vi "lab7_task2.vi"() -> ()   [LabVIEW 2021]
uses:
  <vilib>/DAQmx/write.llb/DAQmx Write (Digital Bool 1Line 1Point).vi
  <vilib>/DAQmx/read.llb/DAQmx Read (Analog Wfm 1Chan NSamp).vi
  <vilib>/DAQmx/create/channels.llb/DAQmx Create Channel (AI-Voltage-Basic).vi
  <vilib>/DAQmx/configure/timing.llb/DAQmx Timing (Sample Clock).vi
  <vilib>/DAQmx/configure/trigger.llb/DAQmx Start Trigger (Digital Edge).vi
  <vilib>/DAQmx/miscellaneous.llb/DAQmx Fill In Error Info.vi
  <vilib>/DAQmx/create/channels.llb/DAQmx Create Channel (DO-Digital Output).vi
panel:
  in  "stop 2":bool
  in  "Trigger \nButton":bool
  in  "stop":bool
  in  "# samples to read":i32=1000
  out "Waveform Graph":waveform(dbl)(graph)
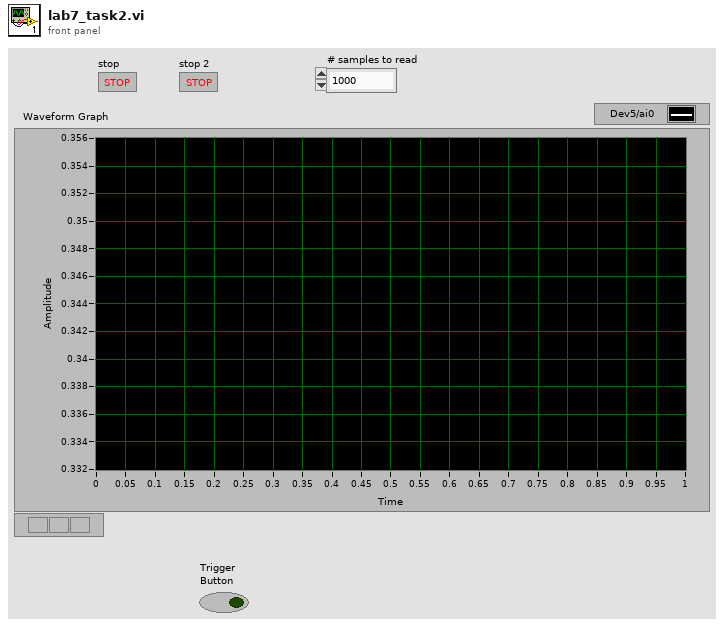
[diagram p1: front panel]
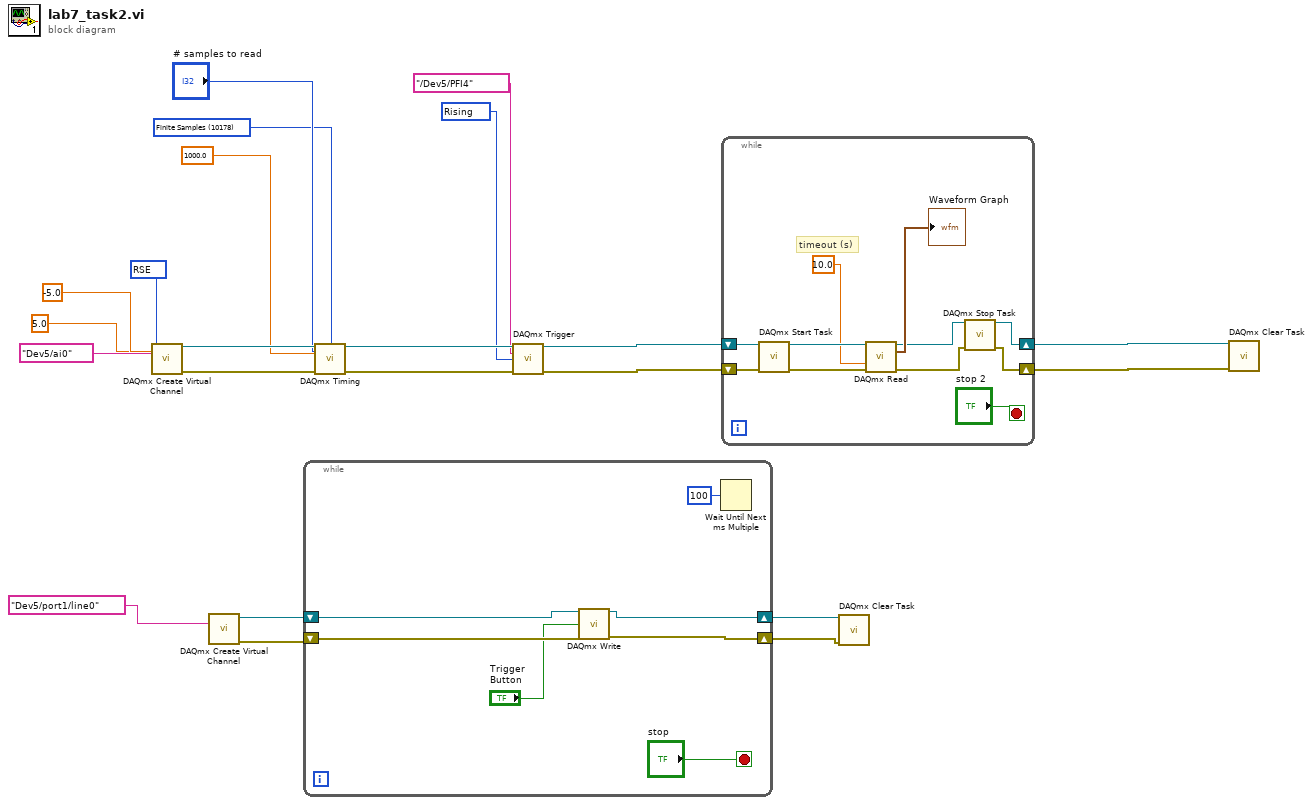
[diagram p0: block diagram]
diagram:
  w11 = 10083 items=["Default"=-1, "RSE"=10083, "NRSE"=10078, "Differential"=10106, "Pseudodifferential"=12529] ("input terminal configuration")
  w12 = 10178 items=["Finite Samples"=10178, "Continuous Samples"=10123, "Hardware Timed Single Point"=12522] ("sample mode")
  w13 = 10280 items=["Rising"=10280, "Falling"=10171] ("edge")
  n1 = call-poly <vilib>:"DAQmx Create Virtual Channel.vi"("maximum value"=5.0, "minimum value"=-5.0, "input terminal configuration"=w11, "physical channels"=tag "Dev5/ai0") -> ("task out"=w18:refnum<k21>, "error out"=w22:errorcluster)  [unwired: 10 in]
  n2 = call-poly <vilib>:"DAQmx Create Virtual Channel.vi"("lines"=tag "Dev5/port1/line0") -> ("task out"=w2:refnum<k21>, "error out"=w3:errorcluster)  [unwired: 13 in]
  n3 = while {
    shift-right: [w27] -> w5
    shift-left: w2 -> [w24]
    shift-right: [w26] -> w4
    shift-left: w3 -> [w25]
    stop <- "stop" stop-if-true
    n4 = call-poly <vilib>:"DAQmx Write.vi"("task/channels in"=w24, "data"="Trigger \nButton", "error in"=w25) -> ("task out"=w27:refnum<k21>, "error out"=w26:errorcluster)  [unwired: 10 in, 1 out]
    n5 = Wait Until Next ms Multiple(millisecond multiple=u32 100) -> ()  [unwired: 1 out]
  }
  n6 = call-poly <vilib>:"DAQmx Timing.vi"("task/channels in"=w18, "sample mode"=w12, "samples per channel"="# samples to read", "rate"=1000.0, "error in"=w22) -> ("task out"=w17:refnum<k21>, "error out"=w21:errorcluster)  [unwired: 9 in]
  n7 = call-poly <vilib>:"DAQmx Trigger.vi"("task/channels in"=w17, "source"=tag "/Dev5/PFI4", "edge"=w13, "error in"=w21) -> ("task out"=w16:refnum<k21>, "error out"=w20:errorcluster)  [unwired: 10 in]
  n8 = while {
    shift-right: [w30] -> w19
    shift-left: w20 -> [w40]
    shift-right: [w32] -> w15
    shift-left: w16 -> [w38]
    stop <- "stop 2" stop-if-true
    # "timeout (s)"
    n9 = call <vilib>:"DAQmx Start Task.vi"("task/channels in"=w38, "error in"=w40) -> ("task out"=w37:refnum<k21>, "error out"=w39:errorcluster)  [unwired: 12 in]
    n10 = call-poly <vilib>:"DAQmx Read.vi"("task/channels in"=w37, "timeout"=10.0, "error in"=w39) -> ("task out"=w33:refnum<k21>, "data"=→"Waveform Graph":waveform(dbl), "error out"=w31:errorcluster)  [unwired: 10 in]
    n11 = call <vilib>:"DAQmx Stop Task.vi"("task/channels in"=w33, "error in"=w31) -> ("task out"=w32:refnum<k21>, "error out"=w30:errorcluster)  [unwired: 12 in]
  }
  n12 = call <vilib>:"DAQmx Clear Task.vi"("task in"=w5, "error in"=w4) -> ()  [unwired: 13 in, 1 out]
  n13 = call <vilib>:"DAQmx Clear Task.vi"("task in"=w15, "error in"=w19) -> ()  [unwired: 13 in, 1 out]
